vi "Output single digital pulse loop.vi"() -> ()   [LabVIEW 2020]
uses:
  <vilib>/DAQmx/create/channels.llb/DAQmx Create Channel (CO-Pulse Generation-Time).vi
  <resource>/objmgr/daqmx.rc
panel:
  out "error out":errorcluster
  in  "Number of pulses":i32=5
  out "elapsed time":dbl
  in  "Pulse Duration":dbl=0.25 format="%.6f"
  in  "Output Terminal":tag="/Dev2/PFI0"
  in  "Counter":tag="Dev2/ctr0"
  in  "Stop":bool
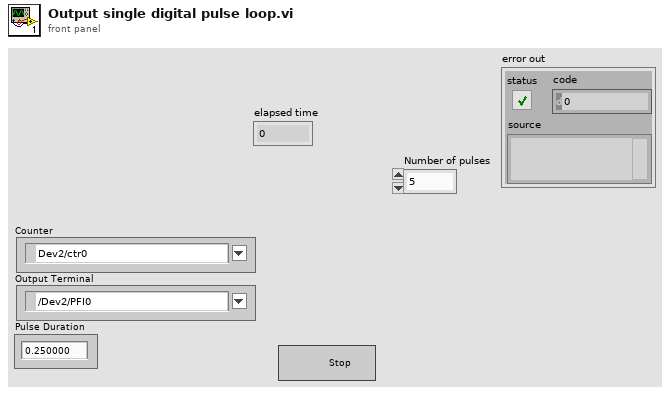
[diagram p1: front panel]
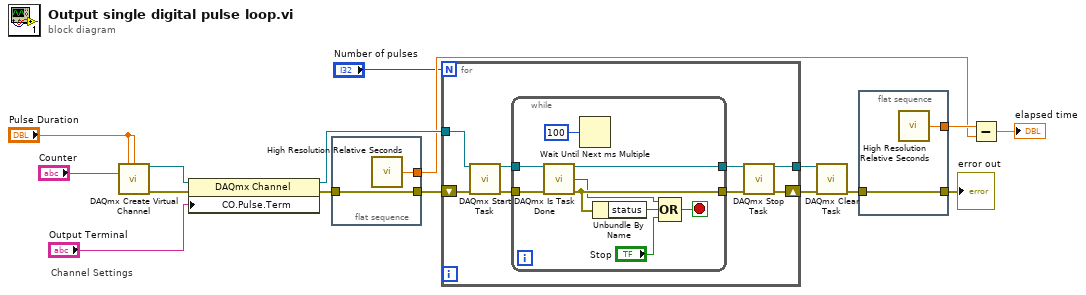
[diagram p0: block diagram]
diagram:
  # "Channel Settings"
  n1 = call-poly <vilib>:"DAQmx Create Virtual Channel.vi"("high time"="Pulse Duration", "low time"="Pulse Duration", "counter"="Counter") -> ("task out"=w15:refnum<k21>, "error out"=w14:errorcluster)  [unwired: 11 in]
  n2 = property class="DAQmx Channel"(reference=w15, error in=w14, "CO.Pulse.Term"="Output Terminal") -> (reference out=w12:refnum<k21>, error out=w10:errorcluster)
  n3 = flat-sequence {
    tunnel: w10 -> [w18]
    tunnel: [w18] -> w9
    tunnel: [w17] -> w7
    frame #0 {
      n4 = call <vilib>:"High Resolution Relative Seconds.vi"() -> ("relative seconds"=w17:dbl)
    }
  }
  n5 = for {
    N: "Number of pulses" -> [_]
    tunnel: w12 -> [w24]
    shift-right: [w19] -> w2
    shift-left: w9 -> [w21]
    tunnel: [w20] -> w4
    n6 = call <vilib>:"DAQmx Start Task.vi"("task/channels in"=w24, "error in"=w21) -> ("task out"=w26:refnum<k21>, "error out"=w25:errorcluster)  [unwired: 12 in]
    n7 = while {
      tunnel: w26 -> [w35]
      tunnel: w25 -> [w34]
      tunnel: [w31] -> w22
      tunnel: [w32] -> w23
      stop <- w33 stop-if-true
      n8 = call <vilib>:"DAQmx Is Task Done.vi"("task/channels in"=w35, "error in"=w34) -> ("task out"=w32:refnum<k21>, "task done?"=w27:bool, "error out"=w31:errorcluster)  [unwired: 11 in]
      n9 = Wait Until Next ms Multiple(millisecond multiple=u32 100) -> ()  [unwired: 1 out]
      n10 = Unbundle By Name(w31) -> ("status"=w30:bool)
      n11 = Compound Arithmetic op=OR(w27, w30, "Stop") -> (w33:bool)
    }
    n12 = call <vilib>:"DAQmx Stop Task.vi"("task/channels in"=w23, "error in"=w22) -> ("task out"=w20:refnum<k21>, "error out"=w19:errorcluster)  [unwired: 12 in]
  }
  n13 = call <vilib>:"DAQmx Clear Task.vi"("task in"=w4, "error in"=w2) -> ("error out"=w3:errorcluster)  [unwired: 13 in]
  n14 = flat-sequence {
    tunnel: w3 -> [w37]
    tunnel: [w37] -> w1
    tunnel: [w36] -> w8
    frame #0 {
      n15 = call <vilib>:"High Resolution Relative Seconds.vi"() -> ("relative seconds"=w36:dbl)
    }
  }
  n16 = Subtract(x=w8, y=w7) -> (x-y=→"elapsed time":dbl)
  "error out" <- w1
